vi "124-Outer Test.vi"(8 "error in":errorcluster) -> (0 "error out":errorcluster)   [LabVIEW 2013]
uses:
  classes/Test/Test.lvclass
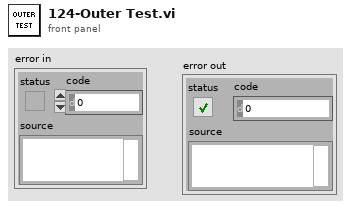
[diagram p1: front panel]
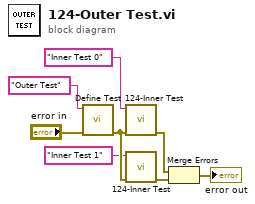
[diagram p0: block diagram]
diagram:
  n1 = call "Define Test.vi"("error in (no error)"="error in", "Label (VI Title)"="Outer Test") -> ("error out"=w7:errorcluster)  [unwired: 9 in]
  n2 = call "124-Inner Test.vi"("error in (no error)"=w7, "Label (VI Title)"="Inner Test 0") -> ("error out"=w6:errorcluster)  [unwired: 9 in]
  n3 = call "124-Inner Test.vi"("error in (no error)"=w7, "Label (VI Title)"="Inner Test 1") -> ("error out"=w5:errorcluster)  [unwired: 9 in]
  n4 = Merge Errors(w6, w5) -> (→"error out":errorcluster)
